vi "test_VI Set-Get Protocol ConvBox.vi"(8 "error in (no error)":errorcluster, 11 "TestCase in":refnum<class "Instrument Addon Scripting API Custom Device Unit Tests.lvclass">) -> (0 "error out":errorcluster, 3 "TestCase out":refnum<class "Instrument Addon Scripting API Custom Device Unit Tests.lvclass">)   [LabVIEW 2018, in "Instrument Addon Scripting API Custom Device Unit Tests.lvclass"]
uses:
  Instrument Addon Scripting API Custom Device Unit Tests.lvclass
  Addon/Support Libraries/Protocols.lvlibp/RS-xxx to GPIB ConvBox/RS-xxx to GPIB ConvBox.lvclass
  C:/Users/nitest/Git/NI VS Instrument Addon Fork/Source/Addon/Support Libraries/Protocols.lvlibp/Protocol Parent/Protocol Parent.lvclass
  NationalInstruments.VeriStand.SystemDefinitionAPI
  Addon/Support Libraries/Protocols.lvlibp/RS-xxx to GPIB ConvBox/Data Access/Write Assert Ren with IFC.vi
  Addon/Support Libraries/Protocols.lvlibp/RS-xxx to GPIB ConvBox/Data Access/Write ConvBox Address.vi
  Addon/Support Libraries/Protocols.lvlibp/RS-xxx to GPIB ConvBox/Data Access/Write GPIB Address.vi
  Addon/Support Libraries/Protocols.lvlibp/RS-xxx to GPIB ConvBox/Data Access/Write IST bit sense.vi
  Addon/Support Libraries/Protocols.lvlibp/RS-xxx to GPIB ConvBox/Data Access/Write Port.vi
  Addon/Support Libraries/Protocols.lvlibp/RS-xxx to GPIB ConvBox/Data Access/Write System controller.vi
  Instrument Addon Scripting API Test Assets/Instrument Addon Scripting API Test Assets.lvclass
  <vilib>/addons/_JKI Toolkits/VI Tester/TestCase.llb/TestCase.lvclass
  APIs/Scripting API/Instrument Addon Scripting API.lvlib
  C:/Program Files (x86)/National Instruments/LabVIEW 2018/vi.lib/addons/_JKI Toolkits/VI Tester/TestCase.llb/TestCase.lvclass
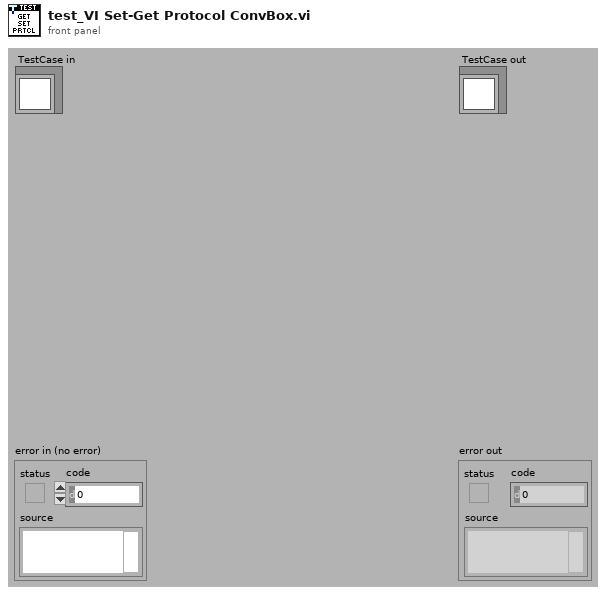
[diagram p1: front panel]
types:
  T1 = typedef "Custom Device API.lvlib/Custom Device Item Ref.ctl" = u64
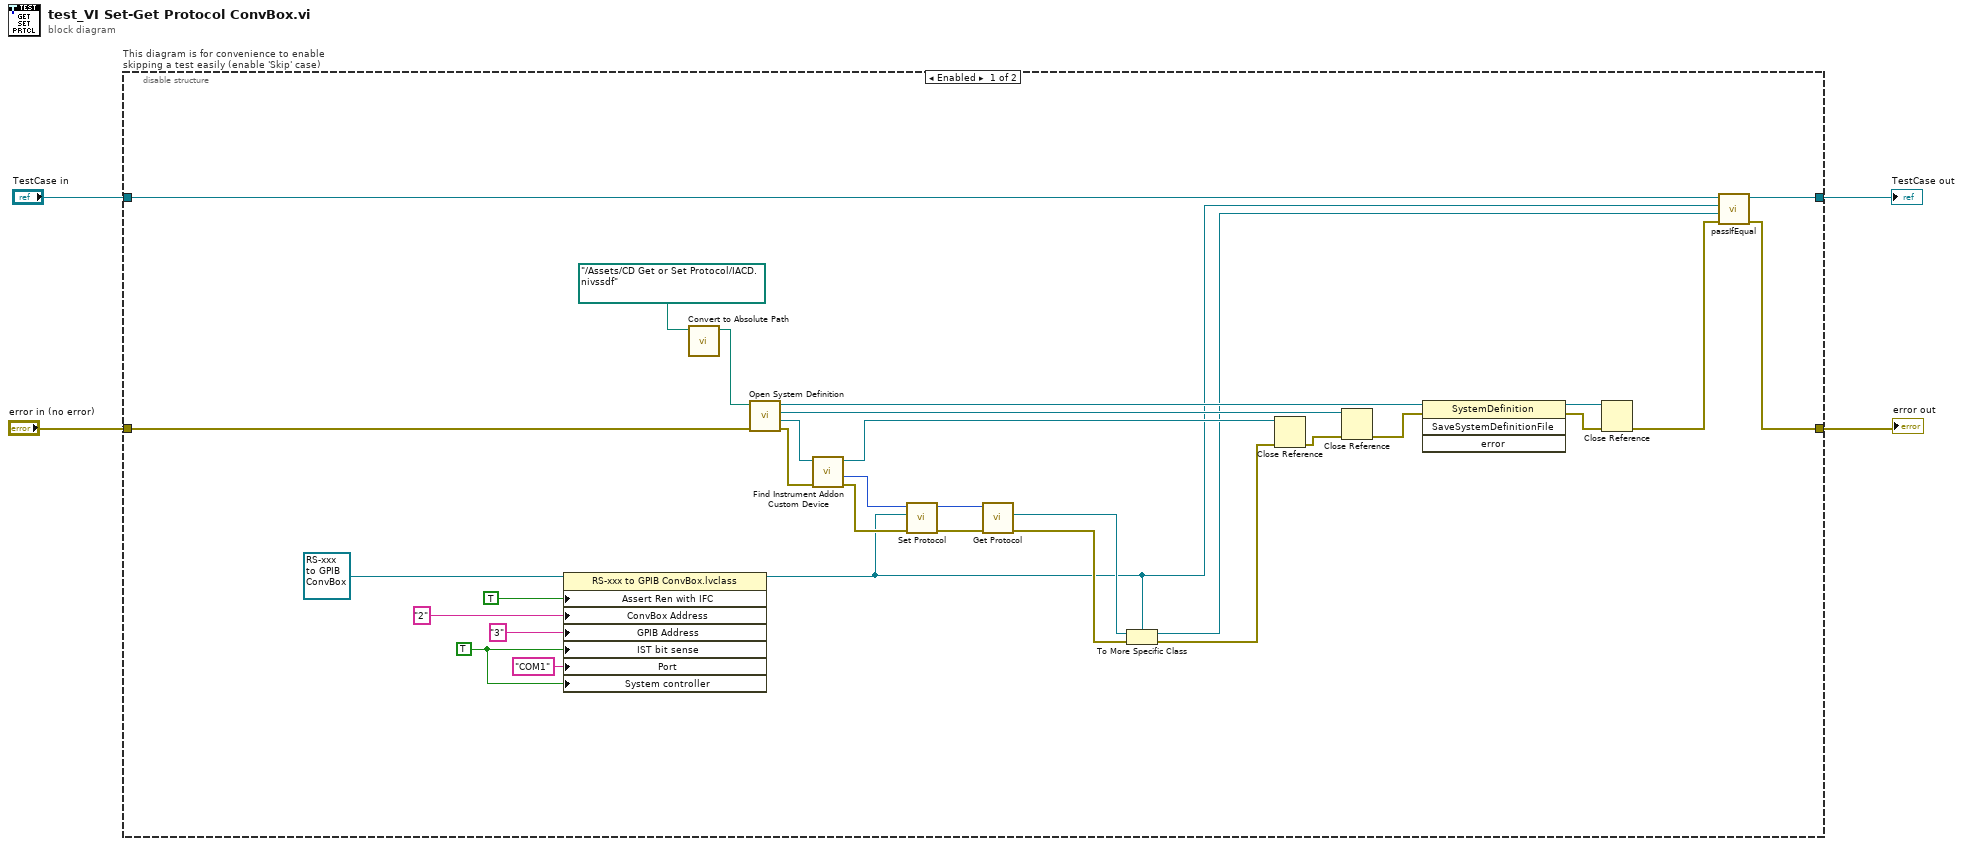
[diagram p0: block diagram]
diagram:
  n1 = disable-structure "This diagram is for convenience to enable skipping a test easily (enable 'Skip' case)" shown="Enabled" {
    disable-tunnel: "TestCase in" -> [w16 w39]
    disable-tunnel: [w15 w37] -> w1
    disable-tunnel: [w11 w38] -> w3
    disable-tunnel: "error in (no error)" -> [w35 w36]
    frame Enabled {
      w5 = TRUE ("Assert Ren with IFC")
      n2 = property class="RS-xxx to GPIB ConvBox.lvclass"(reference=refnum<class "RS-xxx to GPIB ConvBox.lvclass"> refnum ("Protocols.lvlibp:RS-xxx to GPIB ConvBox.lvclass"), "Assert Ren with IFC"=TRUE, "ConvBox Address"="2", "GPIB Address"="3" ("ConvBox Address"), "IST bit sense"=w5, "Port"="COM1", "System controller"=w5) -> (reference out=w13:refnum<class "RS-xxx to GPIB ConvBox.lvclass">)  [unwired: 1 in, 1 out]
      n3 = call "Convert to Absolute Path.vi"("System Definition File"=path "../Assets/CD Get or Set Protocol/IACD.nivssdf" ("SDF file")) -> ("Absolute Path"=w33:path)  [unwired: 10 in]
      n4 = call "Open System Definition.vi"("error in (no error)"=w35, "System Definition File"=w33) -> ("error out"=w30:errorcluster, "Target Refnum"=w29:refnum<k24>, "Root Refnum"=w32:refnum<k24>, "System Definition Refnum"=w23:refnum<k24>)  [unwired: 6 in]
      n5 = call "Find Instrument Addon Custom Device.vi"("error in"=w30, "target in"=w29) -> ("error out"=w28:errorcluster, "NodeID"=w27:u64, "target out"=w26:refnum<k24>)  [unwired: 7 in]
      n6 = call "Set Protocol.vi"("Error In"=w28, "Protocol in"=w13, "Instrument Addon Refnum In"=w27) -> ("Error Out"=w24:errorcluster, "Instrument Addon Refnum Out"=w25:T1)  [unwired: 7 in]
      n7 = call "Get Protocol.vi"("Error In"=w24, "Instrument Addon Refnum In"=w25) -> ("Error Out"=w18:errorcluster, "Protocol"=w19:refnum<class "Protocol Parent.lvclass">)  [unwired: 7 in, 1 out]
      n8 = To More Specific Class(target class=w13, reference=w19, error in=w18) -> (specific class reference=w14:refnum<class "RS-xxx to GPIB ConvBox.lvclass">, error out=w17:errorcluster)
      n9 = Close Reference(reference=w26, error in (no error)=w17) -> (error out=w31:errorcluster)
      n10 = Close Reference(reference=w32, error in (no error)=w31) -> (error out=w22:errorcluster)
      n11 = invoke class="SystemDefinition" method="SaveSystemDefinitionFile"(reference=w23, error in=w22) -> (reference out=w21:refnum<k24>, error out=w20:errorcluster)  [unwired: 2 in, 2 out]
      n12 = Close Reference(reference=w21, error in (no error)=w20) -> (error out=w12:errorcluster)
      n13 = call-dynamic "passIfEqual.vi"("error in (no error)"=w12, "y"=w14, "x"=w13, "TestCase in"=w16) -> ("error out"=w11:errorcluster, "TestCase out"=w15:refnum<class "Instrument Addon Scripting API Custom Device Unit Tests.lvclass">)  [unwired: 6 in]
    }
    frame Disabled {
      # "skip test result while test is under development"
      n14 = call <vilib>:"skip.vi"("error in (no error)"=w36, "TestCase in"=w39) -> ("error out"=w38:errorcluster, "TestCase out"=w37:refnum<class "Instrument Addon Scripting API Custom Device Unit Tests.lvclass">)  [unwired: 8 in]
    }
  }
  "error out" <- w3
  "TestCase out" <- w1
